vi "GUI Monitoring Loop.vi"(8 "error in (no error)":errorcluster, 10 "Sync Objects":T1, 11 "FOFB Parameters":T2) -> (0 "error out":errorcluster)   [LabVIEW 2011, in "User Interface VIs.lvlib"]
uses:
  User Interface VIs.lvlib
  Types Definitions/Type FOFB Parameters.ctl
  Types Definitions/Type Network Configuration.ctl
  Types Definitions/Type FA Configuration.ctl
  Types Definitions/Type Response Matrix Measurement Configuration.ctl
  Types Definitions/Type Correction Algorithm Configuration.ctl
  Types Definitions/Type Acquisition Network Configuration.ctl
  Types Definitions/Type Actuation Network Configuration.ctl
  Types Definitions/Type FOFB GUI.ctl
  Types Definitions/Type Configuration Loop Mode.ctl
  Types Definitions/Type Configuration Data (GUI to Controller).ctl
  Types Definitions/Type Monitoring Data.ctl
  Types Definitions/Type Diagnostics Data.ctl
  Types Definitions/Type CPU Loads Array.ctl
  Types Definitions/Type CPU Loads.ctl
  Types Definitions/Type Diagnostics Sample.ctl
  Types Definitions/Type Monitoring Sample.ctl
  <vilib>/Platform/TimedLoop/XDataNode/timing_clust.ctl
  <vilib>/Platform/TimedLoop/XDataNode/nitl_modes.ctl
  <vilib>/Platform/TimedLoop/XDataNode/wakeup.ctl
  <vilib>/Platform/TimedLoop/XDataNode/XDataNode.xnode
  Type Definitions.lvlib
  <vilib>/Platform/TimedLoop/XDataNode/XDNodeRunTimeDep.lvlib
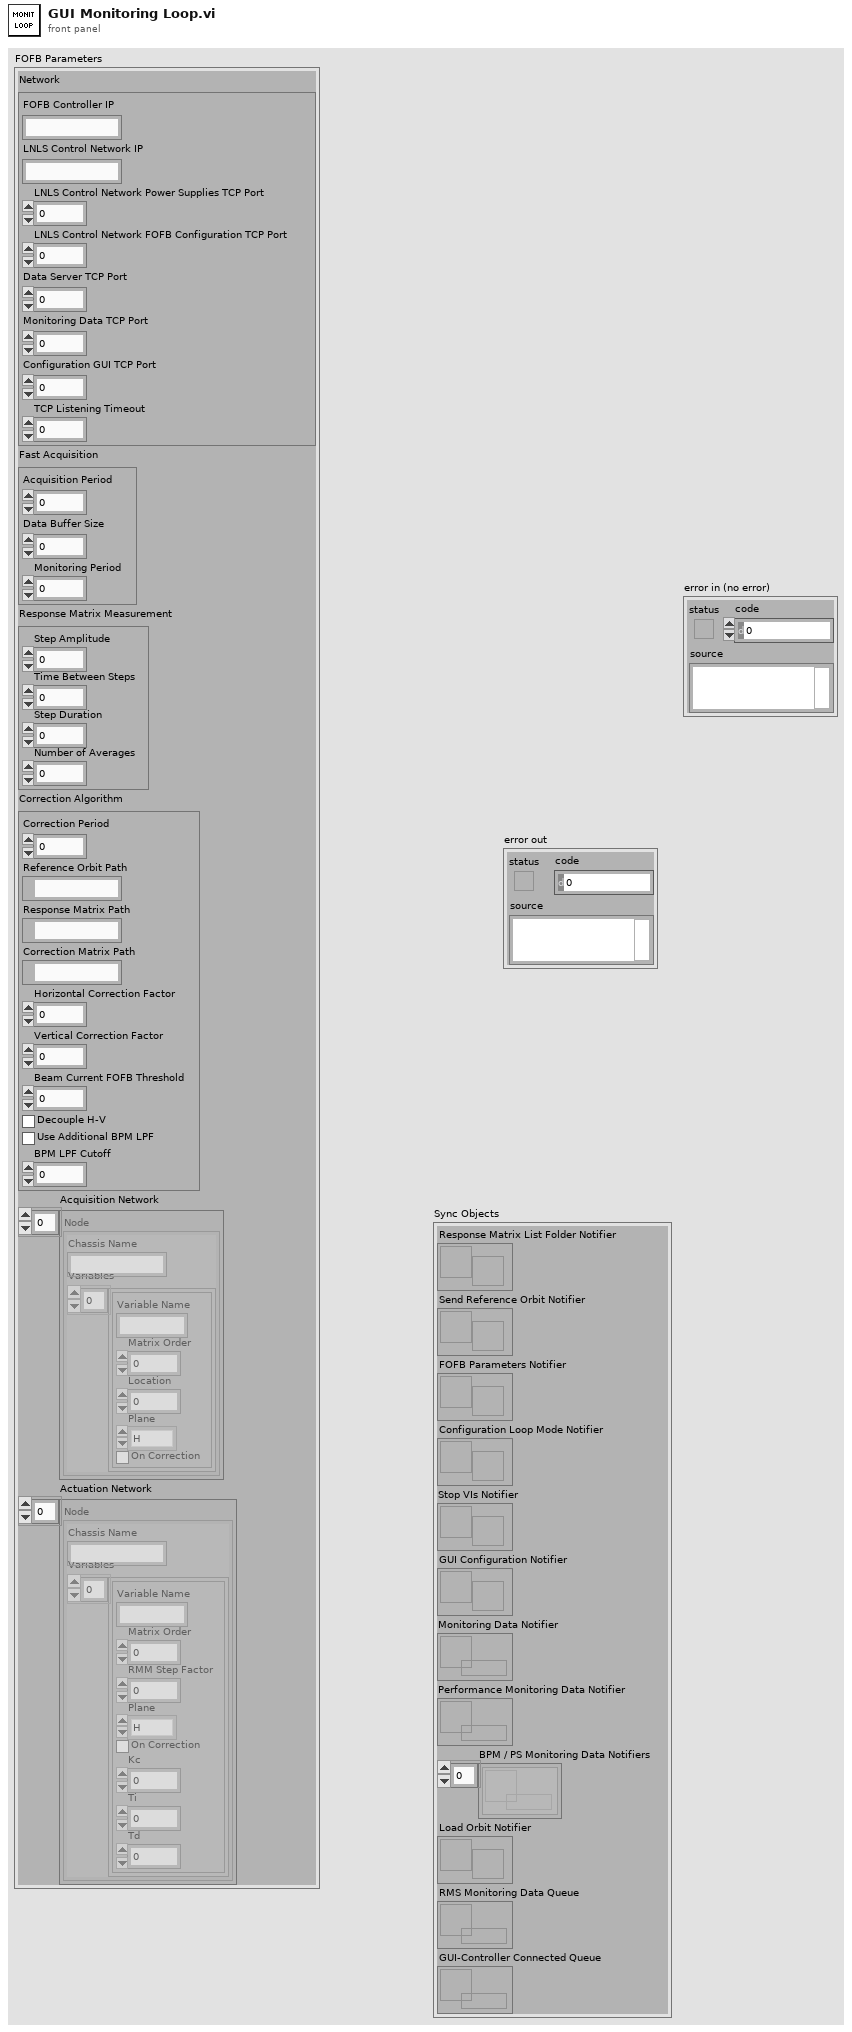
[diagram p1: front panel]
types:
  T1 = typedef "Type Definitions.lvlib/Type FOFB GUI.ctl" = cluster{"Response Matrix List Folder Notifier":refnum<notifier>, "Send Reference Orbit Notifier":refnum<notifier>, "FOFB Parameters Notifier":refnum<notifier>, "Configuration Loop Mode Notifier":refnum<notifier>, "Stop VIs Notifier":refnum<notifier>, "GUI Configuration Notifier":refnum<notifier>, "Monitoring Data Notifier":refnum<queue>, "Performance Monitoring Data Notifier":refnum<queue>, "BPM / PS Monitoring Data Notifiers":refnum<queue>[], "Load Orbit Notifier":refnum<notifier>, "RMS Monitoring Data Queue":refnum<queue>, "GUI-Controller Connected Queue":refnum<queue>}
  T2 = typedef "Type Definitions.lvlib/Type FOFB Parameters.ctl" = cluster{"Network":T3, "Fast Acquisition":T4, "Response Matrix Measurement":T5, "Correction Algorithm":T6, "Acquisition Network":T7, "Actuation Network":T8}
  T3 = typedef "Type Definitions.lvlib/Type Network Configuration.ctl" = cluster{"FOFB Controller IP":string, "LNLS Control Network IP":string, "LNLS Control Network Power Supplies TCP Port":u16, "LNLS Control Network FOFB Configuration TCP Port":u16, "Data Server TCP Port":u16, "Monitoring Data TCP Port":u16, "Configuration GUI TCP Port":u16, "TCP Listening Timeout":i32}
  T4 = typedef "Type Definitions.lvlib/Type FA Configuration.ctl" = cluster{"Acquisition Period":u32, "Data Buffer Size":u32, "Monitoring Period":u32}
  T5 = typedef "Type Definitions.lvlib/Type Response Matrix Measurement Configuration.ctl" = cluster{"Step Amplitude":dbl, "Time Between Steps":u32, "Step Duration":u32, "Number of Averages":u32}
  T6 = typedef "Type Definitions.lvlib/Type Correction Algorithm Configuration.ctl" = cluster{"Correction Period":u32, "Reference Orbit Path":path, "Response Matrix Path":path, "Correction Matrix Path":path, "Horizontal Correction Factor":dbl, "Vertical Correction Factor":dbl, "Beam Current FOFB Threshold":dbl, "Decouple H-V":bool, "Use Additional BPM LPF":bool, "BPM LPF Cutoff":dbl}
  T7 = typedef "Type Definitions.lvlib/Type Acquisition Network Configuration.ctl" = cluster{"Chassis Name":string, "Variables":cluster{"Variable Name":string, "Matrix Order":u32, "Location":dbl, "Plane":enum8{"H", "V"}, "On Correction":bool}[]}[]
  T8 = typedef "Type Definitions.lvlib/Type Actuation Network Configuration.ctl" = cluster{"Chassis Name":string, "Variables":cluster{"Variable Name":string, "Matrix Order":u32, "RMM Step Factor":dbl, "Plane":enum8{"H", "V"}, "On Correction":bool, "Kc":dbl, "Ti":dbl, "Td":dbl}[]}[]
  T9 = enum16{"Idle", "Wait Connection", "Read Data", "Close Connection"}
  T10 = typedef "XDNodeRunTimeDep.lvlib/timing_clust.ctl" = cluster{"Expected End [f-1]":u64, "Actual End [f-1]":u64, "Finished Late? [f-1]":bool, "Expected End [i-1]":u64, "Actual End [i-1]":u64, "Finished Late? [i-1]":bool, "Expected Start [i]":u64, "Actual Start [i]":u64, "Expected Start [f]":u64, "Actual Start [f]":u64, "Source Name":string, "Structure Name":string, "Period":i64, "Deadline":i64, "Offset":i64, "Start":i64, "Priority":i32, "Timeout":i32, "Mode":T11, "Wakeup Reason":T12, "Error":errorcluster, "Source Type":string, "Secondary Source Type":string, "Global End Time":u64, "Global Start Time":u64, "Frame Duration":u64, "Iteration Duration":u64, "Assigned CPU":i32, "I/O Scan Engine Mode":u32}
  T11 = typedef "XDNodeRunTimeDep.lvlib/nitl_modes.ctl" = enum32{"No Change", "Process missed periods, maintain original phase", "Discard missed periods, maintain original phase", "Process missed periods, ignore original phase", "Discard missed periods, ignore original phase"}
  T12 = typedef "XDNodeRunTimeDep.lvlib/wakeup.ctl" = enum32{"Normal", "Aborted", "Asynchronous wakeup", "Timing source error", "Timed loop error", "Timeout"}
  T13 = typedef "Type Definitions.lvlib/Type Monitoring Data.ctl" = cluster{"Timestamp":timestamp, "BPM Readings":dbl[], "PS Readings":dbl[], "PS FOFB Setpoints":dbl[], "PS Status per Rack":u8[], "PS ON-OFF per Rack":u8[], "Operation Mode":enum16{"Idle Mode", "Error Mode", "Manual Mode", "FOFB Mode", "RMM Mode"}, "Diagnostics Data":T14, "Controller Status Table":i32[]}
  T14 = typedef "Type Definitions.lvlib/Type Diagnostics Data.ctl" = cluster{"Time-Critical Loop Missed Iterations":u32, "Time-Critical Loop Execution Time (usec)":u32, "FA Buffer Usage":u32, "Available Memory (bytes)":u32, "CPU Loads Array":T15}
  T15 = typedef "Type Definitions.lvlib/Type CPU Loads Array.ctl" = T16[]
  T16 = typedef "Type Definitions.lvlib/Type CPU Loads.ctl" = cluster{"Total (%)":dbl, "Time Critical (%)":dbl, "Timed Structures (%)":dbl, "High (%)":dbl, "Above Normal (%)":dbl, "Normal (%)":dbl, "Background (%)":dbl, "Idle (%)":dbl, "ISR (%)":dbl}
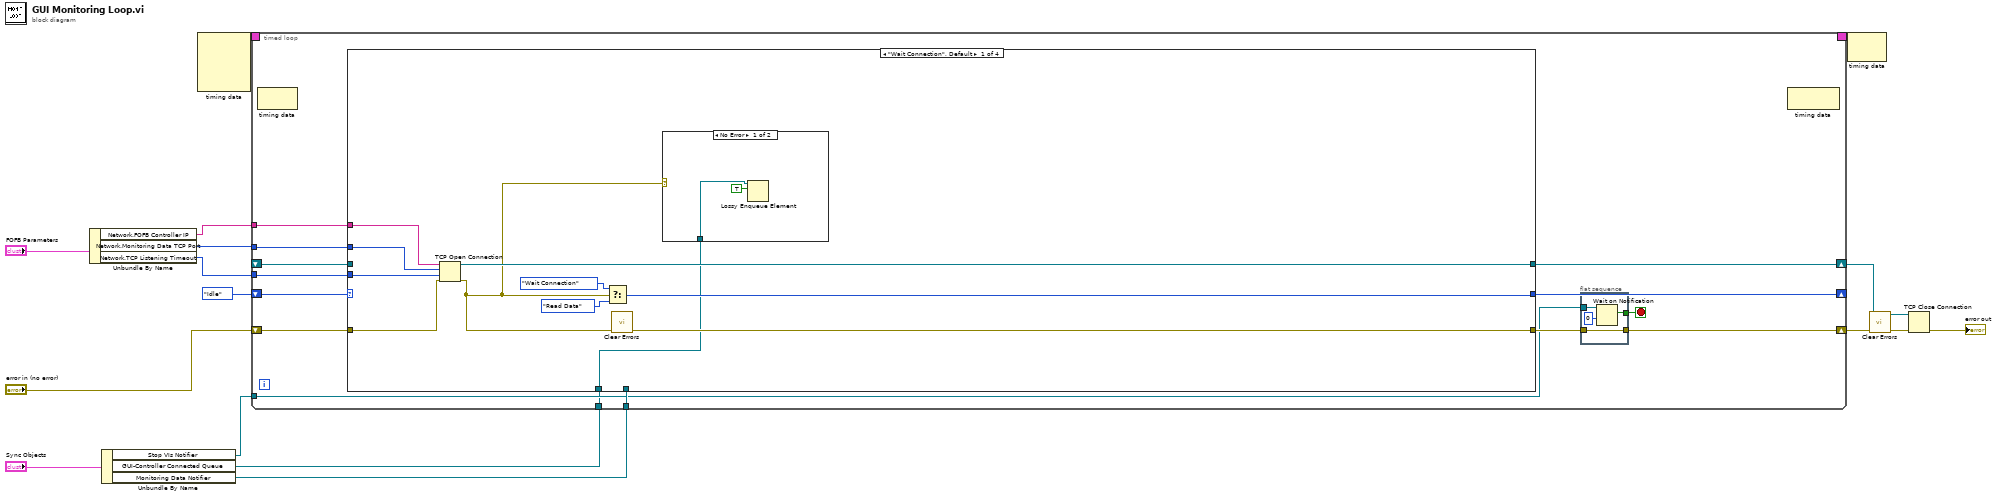
[diagram p0: block diagram]
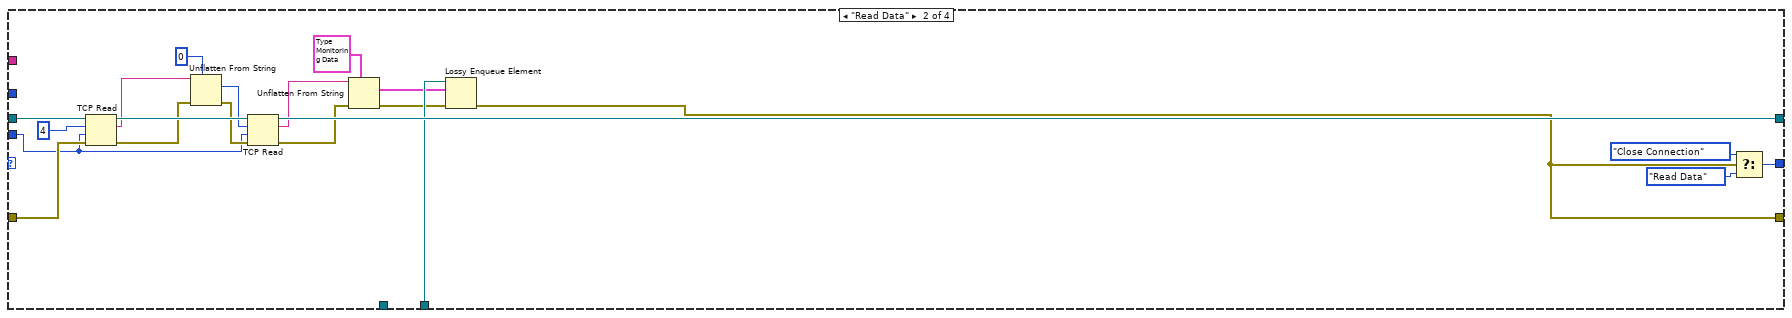
[diagram p3: hidden frame]
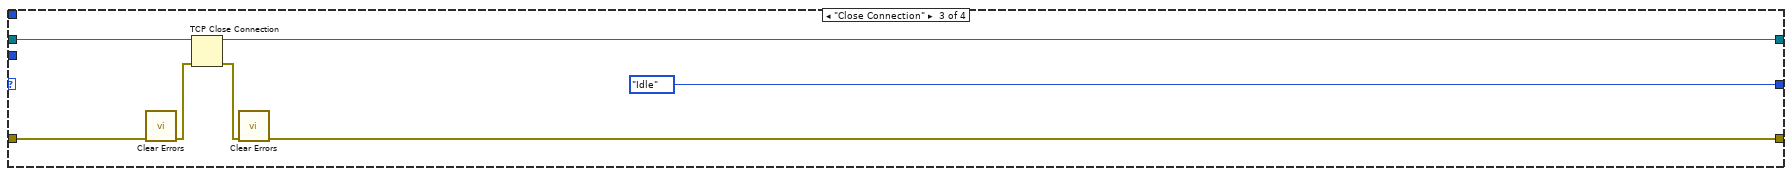
[diagram p4: hidden frame]
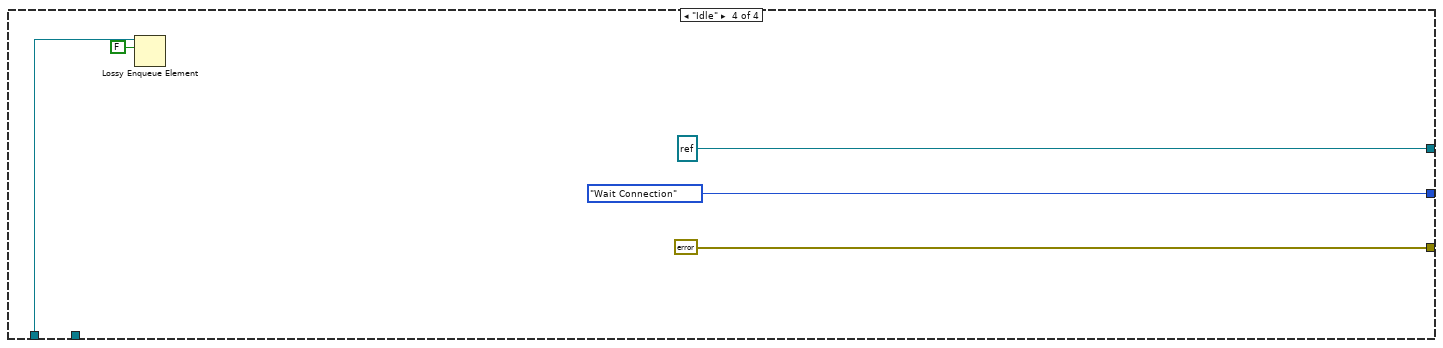
[diagram p5: hidden frame]
diagram:
  n1 = Unbundle By Name("FOFB Parameters") -> ("Network.FOFB Controller IP"=w1:string, "Network.Monitoring Data TCP Port"=w14:u16, "Network.TCP Listening Timeout"=w13:i32)
  n2 = Unbundle By Name("Sync Objects") -> ("Stop VIs Notifier"=w5:refnum<notifier>, "GUI-Controller Connected Queue"=w2:refnum<queue>, "Monitoring Data Notifier"=w4:refnum<queue>)
  n3 = node-c288() -> (w16:T10)  [unwired: 4 in]
  n4 = timed-loop {
    shift-right: [w21] -> w10
    shift-left: "error in (no error)" -> [w30]
    shift-right: [w26] -> _
    shift-left: T9."Idle" ("f") -> [w28]
    shift-right: [w27] -> w11
    shift-left: _ -> [w29]
    tunnel: w4 -> [w25]
    tunnel: w1 -> [w24]
    tunnel: w14 -> [w23]
    tunnel: w13 -> [w22]
    tunnel: w5 -> [w18]
    timing: w16 -> [_]
    timing-out: [_] -> w15
    tunnel: w2 -> [w17]
    stop <- w19 stop-if-true
    n5 = node-c288() -> ()  [unwired: 1 in, 1 out]
    n6 = case shown="\"Wait Connection\", Default" w28 {
      tunnel: [w47 w70 w77 refnum<k5> refnum ("connection ID")] -> w27
      tunnel: [w46 w69 T9."Idle" ("f") T9."Wait Connection" ("f")] -> w26
      tunnel: [w45 w50 w76 errorcluster {"status"=FALSE, "code"=0, "source"=""} ("error out")] -> w20
      tunnel: w30 -> [w44 w66 w71 _]
      tunnel: w29 -> [_ w67 w73 _]
      tunnel: w25 -> [_ w57 _ _]
      tunnel: w24 -> [w41 _ _ _]
      tunnel: w23 -> [w40 _ _ _]
      tunnel: w22 -> [w39 w51 _ _]
      tunnel: w17 -> [w37 _ _ w78]
      frame "Wait Connection", Default {
        n7 = TCP Open Connection(address=w41, remote port or service name=w40, timeout ms (60000)=w39, error in (no error)=w44) -> (connection ID=w47:refnum<k5>, error out=w38:errorcluster)  [unwired: 1 in]
        n8 = Select(t=T9."Wait Connection" ("f"), s=w38, f=T9."Read Data") -> (s? t:f=w46:T9)
        n9 = call <vilib>:"Clear Errors.vi"("error in (no error)"=w38) -> ("error out"=w45:errorcluster)  [unwired: 6 out]
        n10 = case shown="No Error" w38 {
          tunnel: w37 -> [w48 _]
          frame No Error {
            n11 = Lossy Enqueue Element(queue=w48, element=TRUE ("notification")) -> ()  [unwired: 1 in, 4 out]
          }
          frame Error {
          }
        }
      }
      frame "Read Data" {
        n12 = TCP Read(connection ID=w67, bytes to read=4, error in (no error)=w66, 9:w51) -> (connection ID out=w68:refnum<k5>, data out=w62:string, error out=w52:errorcluster)  [unwired: 1 in]
        n13 = Unflatten From String(type=0 ("bytes to read"), binary string=w62, error in (no error)=w52) -> (value=w60:i32, error out=w56:errorcluster)  [unwired: 2 in, 1 out]
        n14 = TCP Read(connection ID=w68, bytes to read=w60, error in (no error)=w56, 9:w51) -> (connection ID out=w70:refnum<k5>, data out=w59:string, error out=w53:errorcluster)  [unwired: 1 in]
        n15 = Unflatten From String(type=T13 {"Timestamp"=timestamp(0 s since 1904-01-01), "BPM Readings"=[], "PS Readings"=[], "PS FOFB Setpoints"=[], "PS Status per Rack"=[], "PS ON-OFF per Rack"=[], "Operation Mode"=enum."Idle Mode", "Diagnostics Data"={"Time-Critical Loop Missed Iterations"=0, "Time-Critical Loop Execution Time (usec)"=0, "FA Buffer Usage"=0, "Available Memory (bytes)"=0, "CPU Loads Array"=[]}, "Controller Status Table"=[]} ("Slow Data"), binary string=w59, error in (no error)=w53) -> (value=w54:T13, error out=w55:errorcluster)  [unwired: 2 in, 1 out]
        n16 = Lossy Enqueue Element(queue=w57, element=w54, error in (no error)=w55) -> (error out=w50:errorcluster)  [unwired: 3 out]
        n17 = Select(t=T9."Close Connection" ("f"), s=w50, f=T9."Read Data") -> (s? t:f=w69:T9)
      }
      frame "Close Connection" {
        n18 = call <vilib>:"Clear Errors.vi"("error in (no error)"=w71) -> ("error out"=w75:errorcluster)  [unwired: 6 in]
        n19 = TCP Close Connection(connection ID=w73, error in (no error)=w75) -> (connection ID out=w77:refnum<k5>, error out=w74:errorcluster)  [unwired: 1 in]
        n20 = call <vilib>:"Clear Errors.vi"("error in (no error)"=w74) -> ("error out"=w76:errorcluster)  [unwired: 6 in]
      }
      frame "Idle" {
        n21 = Lossy Enqueue Element(queue=w78, element=FALSE ("notification")) -> ()  [unwired: 1 in, 4 out]
      }
    }
    n22 = flat-sequence {
      tunnel: [w36] -> w21
      tunnel: w20 -> [w36]
      tunnel: w18 -> [w35]
      tunnel: [w34] -> w19
      frame #0 {
        n23 = Wait on Notification(notifier=w35, timeout in ms (-1)=0) -> (notification=w34:bool)  [unwired: 2 in, 3 out]
      }
    }
    n24 = node-c288() -> ()  [unwired: 1 in, 1 out]
  }
  n25 = node-c288(w15) -> ()  [unwired: 1 out]
  n26 = call <vilib>:"Clear Errors.vi"("error in (no error)"=w10) -> ("error out"=w8:errorcluster)  [unwired: 6 in]
  n27 = TCP Close Connection(connection ID=w11, error in (no error)=w8) -> (error out=→"error out":errorcluster)  [unwired: 1 in, 1 out]
